vi "PostRaw.vi"(0 "InfluxDB in":refnum<class "Client.lvclass">, 5 "Database name":string, 7 "Precision":T1=enum."Nanoseconds", 9 "Content":string, 11 "error in (no error)":errorcluster) -> (4 "InfluxDB out":refnum<class "Client.lvclass">, 15 "error out":errorcluster)   [LabVIEW 2018, in "InfluxDB Client.lvlib" / "Client.lvclass"]
doc: "Creates a database."
uses:
  Client.lvclass
  Controls/Precision.ctl
  InfluxDB Client.lvlib
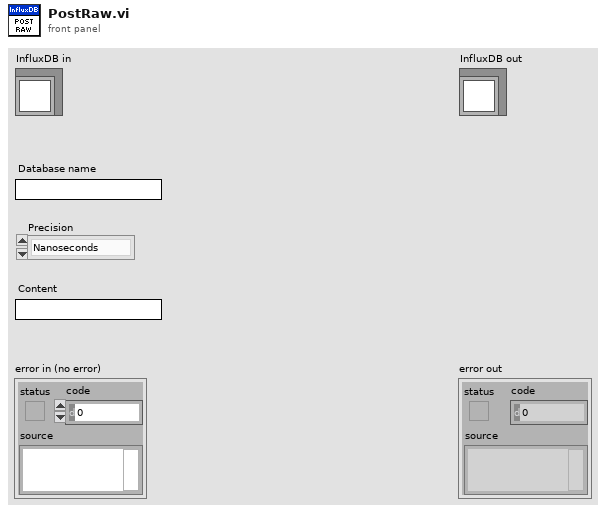
[diagram p1: front panel]
types:
  T1 = typedef "InfluxDB Client.lvlib/Precision.ctl" = enum16{"Seconds", "Milliseconds", "Nanoseconds"}
  T2 = typedef "Dictionary Object RefNum__ogtk.ctl" = refnum<k1>
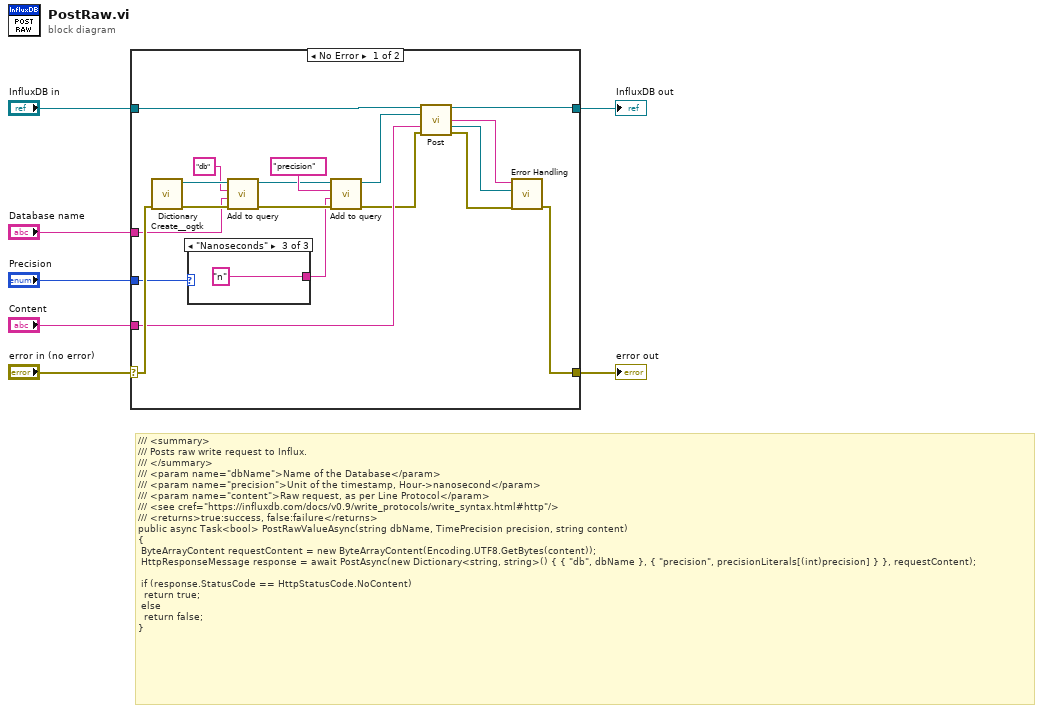
[diagram p0: block diagram]
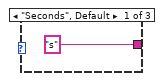
[diagram p2: hidden frame]
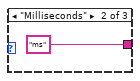
[diagram p3: hidden frame]
diagram:
  # "/// <summary>\n/// Posts raw write request to Influx.\n/// </summary>\n/// <param name=\"dbName\">Name of the Database</param>\n/// <param name=\"precision\">Unit of the timestamp, Hour->nanosecond</param>\n/// <param name=\"content\">Raw request, as per Line Protocol</param>\n/// <see cref=\"https://influxdb.com/docs/v0.9/write_protocols/write_syntax.html#http\"/>\n/// <returns>true:success, false:failure</returns>\npublic async Task<bool> PostRawValueAsync(string dbName, TimePrecision precision, string content)\n{\n\tByteArrayContent requestContent = new ByteArrayContent(Encoding.UTF8.GetBytes(content));\n\tHttpResponseMessage response = await PostAsync(new Dictionary<string, string>() { { \"db\", dbName }, { \"precision\", precisionLiterals[(int)precision] } }, requestContent);\n\n\tif (response.StatusCode == HttpStatusCode.NoContent)\n\t\treturn true;\n\telse\n\t\treturn false;\n}"
  n1 = case shown="No Error" "error in (no error)" {
    selector: "error in (no error)" -> [w22 w31]
    tunnel: [w10 w31] -> w6
    tunnel: [w25 w30] -> w4
    tunnel: "InfluxDB in" -> [w26 w30]
    tunnel: "Database name" -> [w20 _]
    tunnel: "Content" -> [w15 _]
    tunnel: "Precision" -> [w14 _]
    frame No Error {
      n2 = call <userlib>:"Dictionary Create__ogtk.vi"("error in (no error)"=w22) -> ("error out"=w21:errorcluster, "dictionary out"=w24:T2)  [unwired: 9 in]
      n3 = case shown="\"Nanoseconds\"" w14 {
        tunnel: ["s" ("String") "ms" ("String") "n" ("String")] -> w16
        frame "Seconds", Default {
        }
        frame "Milliseconds" {
        }
        frame "Nanoseconds" {
        }
      }
      n4 = call "Add to query.vi"("error in (no error)"=w21, "Value"=w20, "Parameter"="db" ("String"), "Query in"=w24) -> ("error out"=w18:errorcluster, "Query out"=w17:T2)  [unwired: 6 in]
      n5 = call "Add to query.vi"("error in (no error)"=w18, "Value"=w16, "Parameter"="precision" ("String"), "Query in"=w17) -> ("error out"=w12:errorcluster, "Query out"=w13:T2)  [unwired: 6 in]
      n6 = call "Post.vi"("InfluxDB Client in"=w26, "Query"=w13, "buffer"=w15, "error in (no error)"=w12) -> ("InfluxDB Client out"=w25:refnum<class "Client.lvclass">, "Status code"=w9:string, "Headers"=w8:T2, "error out"=w11:errorcluster)  [unwired: 7 in, 1 out]
      n7 = call "Error Handling.vi"("error in (no error)"=w11, "HTTP headers"=w8, "HTTP status code"=w9) -> ("error out"=w10:errorcluster)  [unwired: 8 in]
    }
    frame Error {
    }
  }
  "error out" <- w6
  "InfluxDB out" <- w4
